vi "Initialize.vi"(5 "Password":string, 7 "Username":string, 8 "error in (no error)":errorcluster, 10 "Address":string, 11 "File Transfer Behavior in":refnum<class "File Transfer Behavior.lvclass">) -> (0 "error out":errorcluster, 3 "File Transfer Behavior out":refnum<class "File Transfer Behavior.lvclass">)   [LabVIEW 2015, in "RT Management.lvlib" / "File Transfer Behavior.lvclass"]
doc: "Initializes a specific file transfer protocol session for the given target based upon the specific implementation class passed in."
uses:
  File Transfer Behavior.lvclass
  RT Management.lvlib
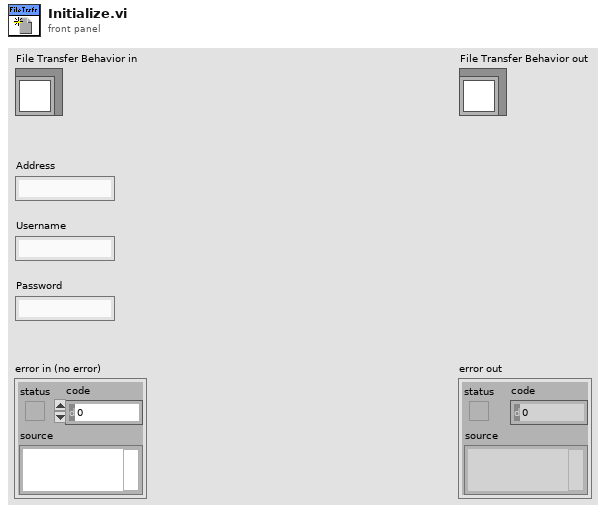
[diagram p1: front panel]
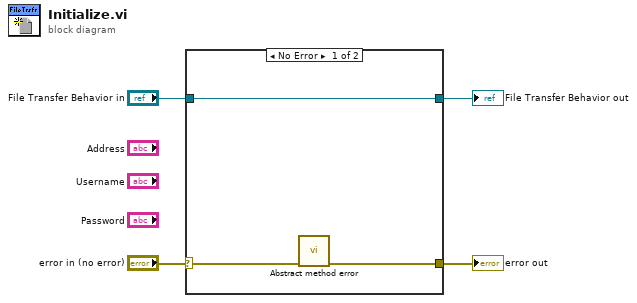
[diagram p0: block diagram]
diagram:
  n1 = case shown="No Error" "error in (no error)" {
    selector: "error in (no error)" -> [w6 w9]
    tunnel: [w5 w9] -> w3
    tunnel: [w7 w8] -> w1
    tunnel: "File Transfer Behavior in" -> [w7 w8]
    frame No Error {
      n2 = call "Abstract method error.vi"("error in (no error)"=w6) -> ("error out"=w5:errorcluster)  [unwired: 10 in]
    }
    frame Error {
    }
  }
  "error out" <- w3
  "File Transfer Behavior out" <- w1
